vi "Close.vi"(8 "error in (no error)":errorcluster, 11 "uService Template in":refnum<class "Tamer.lvclass">) -> (0 "error out":errorcluster, 3 "uService Template out":refnum<class "Tamer.lvclass">)   [LabVIEW 2020, in "Tamer.lvlib" / "Tamer.lvclass"]
uses:
  Tamer.lvclass
  Ancestor/Ancestor/Infinite Message Selector.ctl
  Tamer Consumer Case Selector.ctl
  Ancestor/Ancestor/Ancestor.lvclass
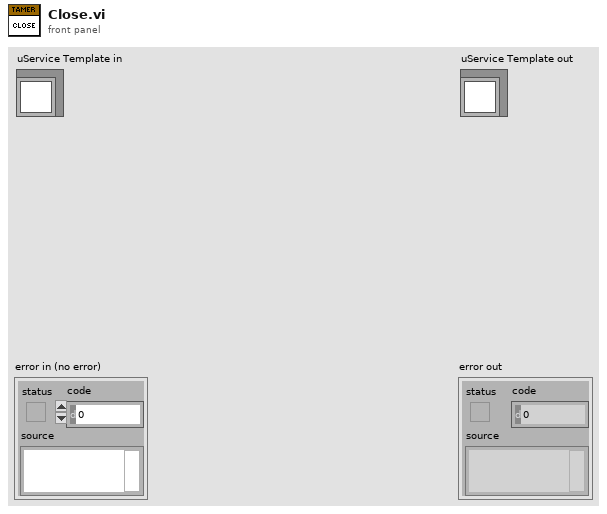
[diagram p1: front panel]
types:
  T1 = typedef "Tamer.lvlib/Tamer.lvclass/Tamer Consumer Case Selector.ctl" = enum16{"New schedule", "Initiate RUN", "Parse Schedules", "Script Checker", "Banana after Quality Check", "Update Crit Lvl", "Propagate Banana", "Reply from Guardian", "Reply from uService", "Timeout of RUN", "uService Replies Check", "Update from Monkey", "Monkey Died", "Reschedule", "Rerun", "Stop DAQ", "Stop Schedule", "Skip Run", "Kill Process", "Update GV"}
  T2 = typedef "TALOS.lvlib/Ancestor.lvlib/Ancestor.lvclass/Infinite Message Selector.ctl" = enum16{"Start", "Stop", "Check", "Flush (Stop all)", "Init"}
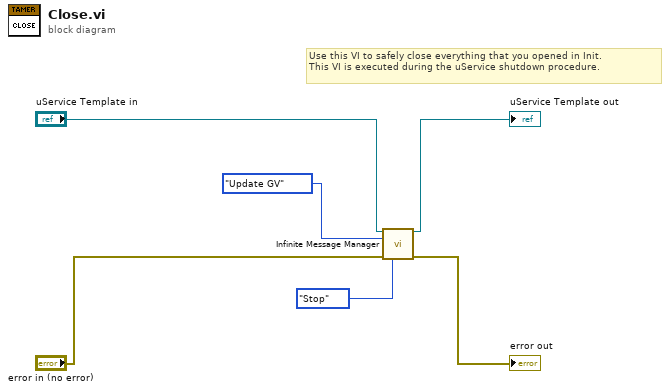
[diagram p0: block diagram]
diagram:
  # "Use this VI to safely close everything that you opened in Init.\nThis VI is executed during the uService shutdown procedure."
  n1 = call-dynamic "Infinite Message Manager.vi"("Father of all uServices in"="uService Template in", "Consumer Case Selector"=Tamer_Consumer_Case_Selector."Update GV" ("Monkey Consumer Case Selector"), "error in (no error)"="error in (no error)", "Infinite Message Selector"=Infinite_Message_Selector."Stop") -> ("Father of all uServices out"=→"uService Template out":refnum<class "Tamer.lvclass">, "error out"=→"error out":errorcluster)  [unwired: 9 in, 1 out]
